vi "Close.vi"(8 "error in (no error)":errorcluster, 11 "Lambda Gen LAN in":refnum<class "Lambda Gen LAN.lvclass">) -> (0 "error out":errorcluster, 3 "Lambda Gen LAN out":refnum<class "Lambda Gen LAN.lvclass">)   [LabVIEW 2025, in "Power Supply.lvlib" / "Lambda Gen LAN.lvclass"]
uses:
  Lambda Gen LAN.lvclass
  Lambda Gen LAN.lvclass/Lambda Gen LAN.ctl
  PS Instrument/Power Supply Instrument.lvclass
  <instrlib>/TDK-Lambda GEN LAN Series/TDK-Lambda GEN LAN Series.lvlib
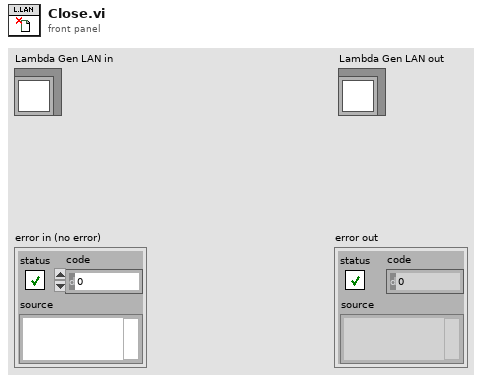
[diagram p1: front panel]
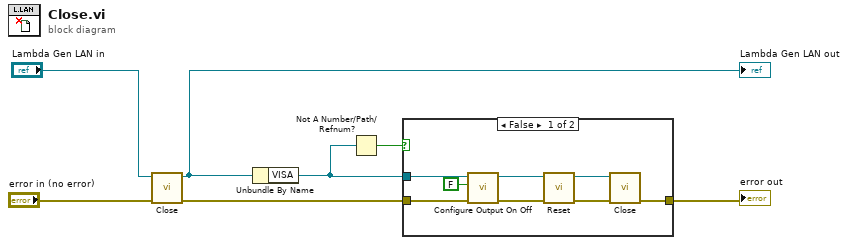
[diagram p0: block diagram]
diagram:
  n1 = call-parent <instrlib>:"Close.vi"("error in (no error)"="error in (no error)", "Power Supply Instrument in"="Lambda Gen LAN in") -> ("error out"=w3:errorcluster, "Power Supply Instrument out"=w1:refnum<class "Lambda Gen LAN.lvclass">)  [unwired: 8 in]
  "Lambda Gen LAN out" <- w1
  n2 = Unbundle By Name(w1) -> ("VISA"=w5:refnum<visa-resource-name>)
  n3 = Not A Number/Path/Refnum?(number/path/refnum=w5) -> (NaN/Path/Refnum?=w4:bool)
  n4 = case shown="False" w4 {
    tunnel: [w13 w16] -> w7
    tunnel: w3 -> [w10 w16]
    tunnel: w5 -> [w12 _]
    frame False {
      n5 = call <instrlib>:"Configure Output On Off.vi"("error"=w10, "Output ON"=FALSE, "VISA"=w12) -> ("error out"=w9:errorcluster, "VISA out"=w11:refnum<visa-resource-name>)  [unwired: 7 in]
      n6 = call <instrlib>:"Reset.vi"("error"=w9, "VISA"=w11) -> ("error out"=w14:errorcluster, "VISA out"=w15:refnum<visa-resource-name>)  [unwired: 8 in]
      n7 = call <instrlib>:"Close.vi"("error"=w14, "VISA name"=w15) -> ("error out"=w13:errorcluster)  [unwired: 9 in]
    }
    frame True {
    }
  }
  "error out" <- w7
